vi "Record Call.vi"(10 "VI Call":refnum<class "VI Call.lvclass">, 11 "One In":refnum<class "Exactly.lvclass">) -> (3 "One Out":refnum<class "Exactly.lvclass">)   [LabVIEW 2020, in "Deprecated Exactly.lvlib" / "Exactly.lvclass"]
uses:
  Exactly.lvclass
  Core/VI Call/VI Call.lvclass
  Exactly.lvclass/Exactly.ctl
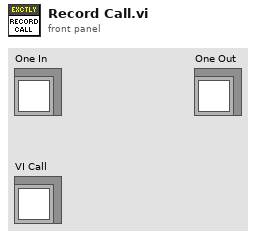
[diagram p1: front panel]
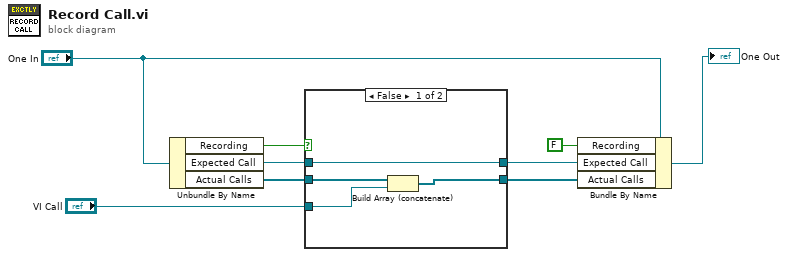
[diagram p0: block diagram]
diagram:
  n1 = Unbundle By Name("One In") -> ("Recording"=w7:bool, "Expected Call"=w1:refnum<class "VI Call.lvclass">, "Actual Calls"=w3:refnum<class "VI Call.lvclass">[])
  n2 = case shown="False" w7 {
    tunnel: "VI Call" -> [w12 w14]
    tunnel: [w10 w14] -> w4
    tunnel: w3 -> [w13 w15]
    tunnel: [w11 w15] -> w2
    tunnel: w1 -> [w10 _]
    frame False {
      n3 = Build Array (concatenate)(w13, w12) -> (w11:refnum<class "VI Call.lvclass">[])
    }
    frame True {
    }
  }
  n4 = Bundle By Name(cluster="One In", "Recording"=FALSE, "Expected Call"=w4, "Actual Calls"=w2) -> (→"One Out":refnum<class "Exactly.lvclass">)
